vi "XML Script - Append Terminal Name (While Condition).vi"(1 "while_loop":string) -> (0 "while_loop.Test Condition":string)   [LabVIEW 2017]
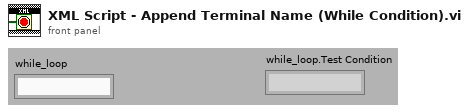
[diagram p1: front panel]
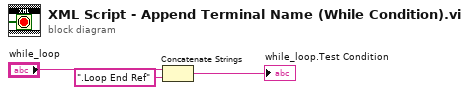
[diagram p0: block diagram]
diagram:
  n1 = Concatenate Strings("while_loop", ".Loop End Ref" ("string")) -> (→"while_loop.Test Condition":string)
